vi "SendCMD.vi"(8 "error in (no error)":errorcluster, 10 "Vision_Modes":T2=enum."ResetCamera") -> (0 "error out":errorcluster)   [LabVIEW 2017, in "VisionHW.lvlib"]
uses:
  VisionHW.lvlib
  TypeDefs/ENUM_Vision_Commands.ctl
  <vilib>/Rock Robotics/WPI/SerialPort/WPI_SerialPortRef.ctl
panel:
  out "SerialPortRef 2":T1
  in  "SerialPortRef":T1
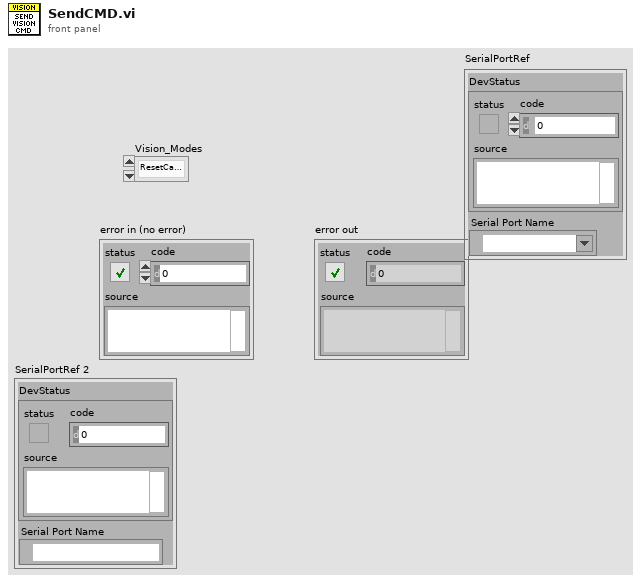
[diagram p1: front panel]
types:
  T1 = typedef "WPI_SerialPortRef.ctl" = cluster{"DevStatus":errorcluster, "Serial Port Name":refnum<visa-resource-name>}
  T2 = typedef "ENUM_Vision_Commands.ctl" = enum16{"Init", "NoOp", "ResetCamera", "VideoOn", "VideoOff", "CubeDetection", "RoadNavigation"}
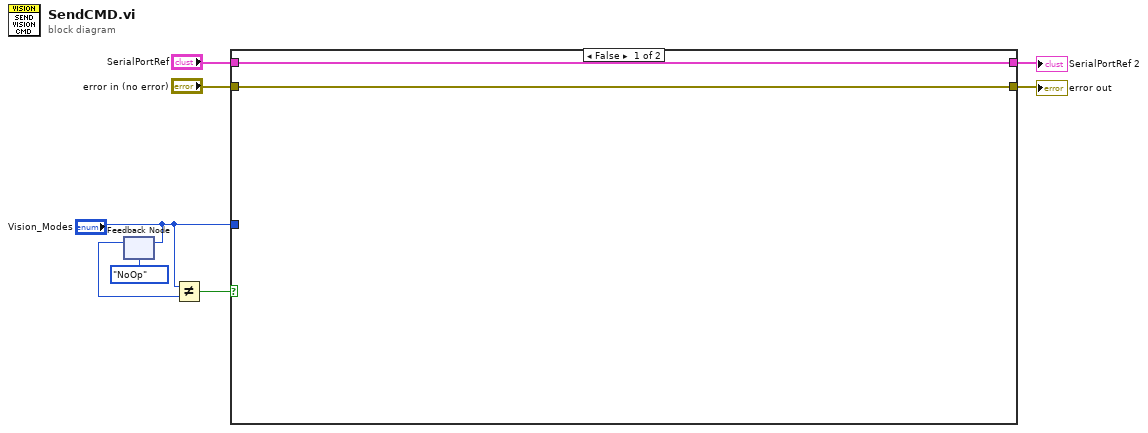
[diagram p0: block diagram]
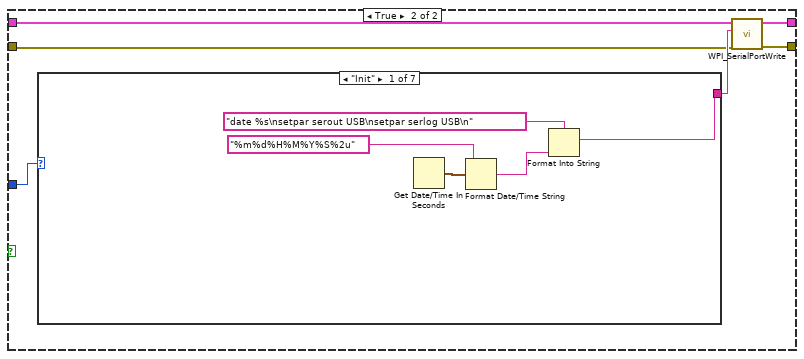
[diagram p2: hidden frame]
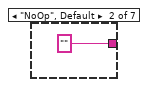
[diagram p3: hidden frame]
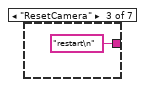
[diagram p4: hidden frame]
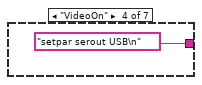
[diagram p5: hidden frame]
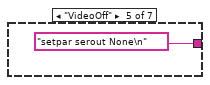
[diagram p6: hidden frame]
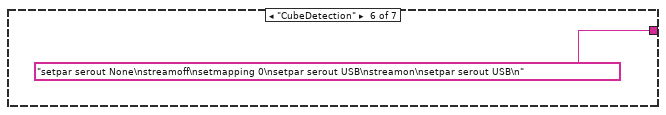
[diagram p7: hidden frame]
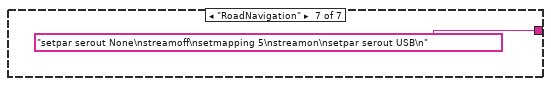
[diagram p8: hidden frame]
diagram:
  n1 = feedback-in #1("Vision_Modes") -> ()
  n2 = feedback #1(ENUM_Vision_Commands."NoOp" ("Vision_Modes")) -> (w7:T2)
  n3 = Not Equal?(x="Vision_Modes", y=w7) -> (x != y?=w5:bool)
  n4 = case shown="False" w5 {
    tunnel: "Vision_Modes" -> [_ w16]
    tunnel: [w9 w14] -> w1
    tunnel: "error in (no error)" -> [w10 w11]
    tunnel: [w10 w15] -> w3
    tunnel: "SerialPortRef" -> [w9 w12]
    frame False {
    }
    frame True {
      n5 = case shown="\"Init\"" w16 {
        tunnel: [w17 "" "restart\n" "setpar serout USB\n" "setpar serout None\n" "setpar serout None\nstreamoff\nsetmapping 0\nsetpar serout USB\nstreamon\nsetpar serout USB\n" "setpar serout None\nstreamoff\nsetmapping 5\nstreamon\nsetpar serout USB\n"] -> w13
        frame "Init" {
          n6 = Get Date/Time In Seconds() -> (seconds since 1Jan1904=w21:timestamp)
          n7 = Format Date/Time String(time format string (%c)="%m%d%H%M%Y%S%2u", seconds (now)=w21) -> (date/time string=w18:string)  [unwired: 1 in]
          n8 = Format Into String(format string="date %s\nsetpar serout USB\nsetpar serlog USB\n" ("write buffer"), w18) -> (resulting string=w17:string)  [unwired: 2 in, 1 out]
        }
        frame "NoOp", Default {
        }
        frame "ResetCamera" {
        }
        frame "VideoOn" {
        }
        frame "VideoOff" {
        }
        frame "CubeDetection" {
        }
        frame "RoadNavigation" {
        }
      }
      n9 = call <vilib>:"WPI_SerialPortWrite.vi"("error in (no error)"=w11, "Buffer"=w13, "SerialPortRef"=w12) -> ("error out"=w15:errorcluster, "SerialPortRef"=w14:T1)  [unwired: 6 in, 1 out]
    }
  }
  "error out" <- w3
  "SerialPortRef 2" <- w1
